vi "浊度电极校准.vi"() -> ()   [LabVIEW 2016, in "斯坦道多参数.lvlib"]
uses:
  <vilib>/Utility/miscctls.llb/LVPointTypeDef.ctl
  <vilib>/Utility/miscctls.llb/LVPositionTypeDef.ctl
  <vilib>/Analysis/NI_AALBase.lvlib
panel:
  out "滤波设定":dbl
  in  "刷新按钮":bool
  out "第三点信号值":dbl
  out "第二点信号值":dbl
  out "第一点信号值":dbl
  out "温度":dbl format="%#.2f"
  out "通讯状态":string
  out "电极状态标志":u16(ring) items=["OK"=0, "第一点校正通过"=1, "第二点校正通过"=2, "悬浮物两点校准第一点校正通过"=11, "悬浮物两点校准第二点校正通过"=12, "浊度三点校正第一点校正通过"=31, "浊度三点校正第二点校正通过"=32, "浊度三点校正第三点校正通过"=33]
  out "第三点校准值":dbl
  out "标液3":dbl
  out "第二点校准值":dbl
  out "第一点校准值":dbl
  in  "校准停止":bool
  in  "校准启动":bool
  in  "校准模式":u16(ring) items=["两点校准", "单点校准", "三点校准"]
  out "最小值":sgl format="%#.2f"
  out "最大值":sgl format="%#.2f"
  out "波形图表":sgl(graph) caption="历史曲线"
  out "mean":dbl caption="均值" format="%#.2f"
  out "standard deviation":dbl caption="标准差" format="%#.2f"
  out "变异系数":dbl format="%#.6f"
  out "测量值":dbl format="%#.2f"
  out "提示":string
  out "标液2":dbl
  out "标液1":dbl
  out "信号值":dbl format="%#.2f"
  out "偏移值补偿":dbl caption="浊度偏移修正值" format="%#.2f"
  out "电极斜率":dbl format="%#.6f"
  out "电极零点":dbl format="%#.6f"
  # "浊度电极设定"
  # "℃"
  # "NTU"
  # "%"
  # "请选择校准模式:"
  # "NTU"
  # "NTU"
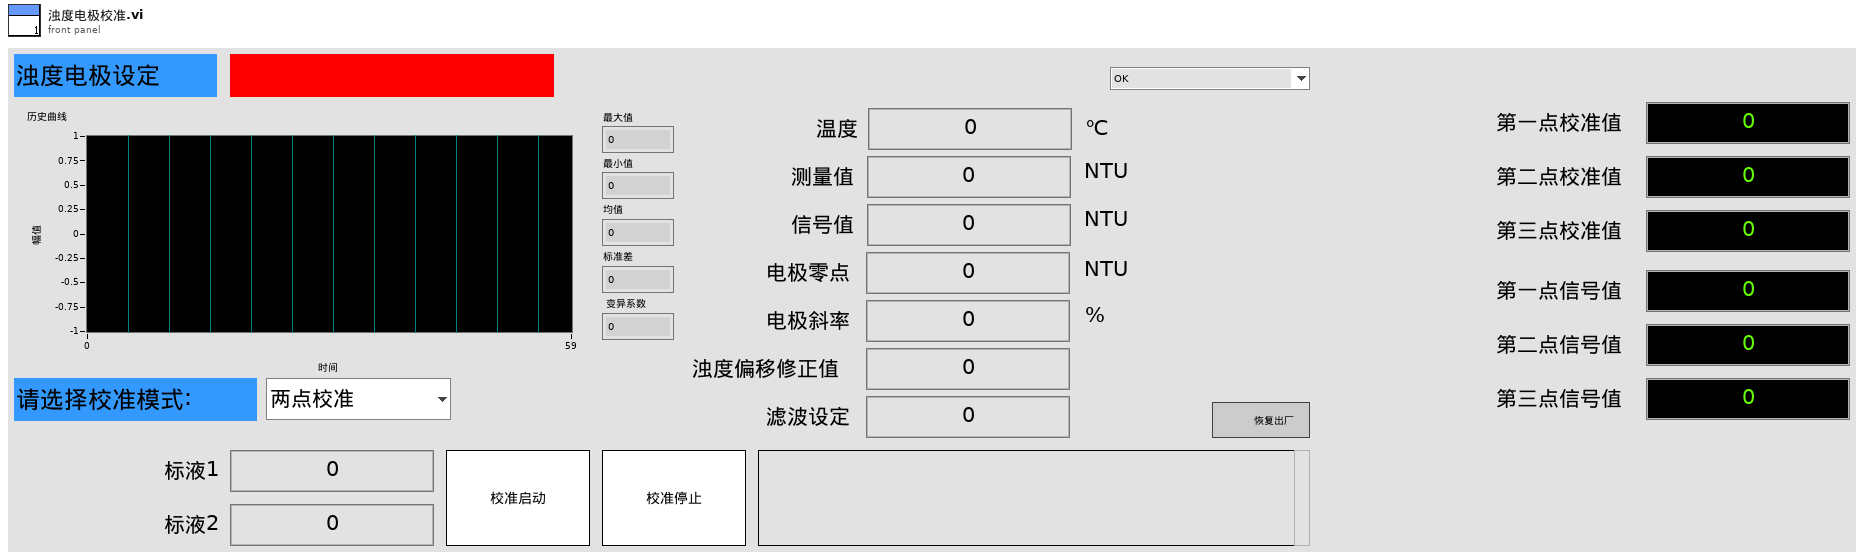
[diagram p1: front panel]
types:
  T1 = enum16{"pH", "DO", "Cond", "Turb", "ORP", "叶绿素a", "藻密度"}
  T2 = typedef "LVPointTypeDef.ctl" = cluster{"Horizontal":i16, "Vertical":i16}
  T3 = cluster{"电极状态标志":u16, "电极型号标志":u16, "浊度测量值":sgl, "温度测量值":sgl, "浊度信号值":sgl, "浊度偏移修正值":sgl, "温度偏移修正值":sgl, "手动温度补偿值":sgl, "浊度电极零点":sgl, "浊度电极斜率":sgl, "第1点标准值记录":sgl, "第1点信号值记录":sgl, "第1点温度值记录":sgl, "第2点标准值记录":sgl, "第2点信号值记录":sgl, "第2点温度值记录":sgl, "命令滤波设定":u16, "温度模式":enum16{"ATC", "MTC"}, "生产批次":u16, "电极序号":u16, "串口地址":u16, "串口波特率":enum16{"9600", "19200", "115200"}, "串口校验位":enum16{"NONE", "ODD", "EVEN"}, "串口停止位":enum16{"1bit", "2bit"}, "第一点标准值":sgl, "第二点标准值":sgl, "第三点标准值":sgl}
  T4 = typedef "LVPositionTypeDef.ctl" = cluster{"Left":i32, "Top":i32}
  T5 = enum8{"Enabled", "Disabled", "Disabled and Grayed Out"}
  T6 = cluster{"测量量程":dbl, "测量精度":dbl, "测量间隔":dbl, "消解温度":dbl, "消解时长":dbl, "空白校准时间":timestamp, "曲线截距":dbl, "曲线斜率":dbl, "测量检出限":dbl, "测量信号值":dbl, "线性相关系数":dbl, "二次多项式系数":dbl, "标样校准时间":timestamp, "稀释倍数":dbl, "三项式系数":dbl, "空白标定系数":dbl, "量程系数":dbl, "F0/ORPA":dbl, "F1/ORPB":dbl, "F2/ORPK":dbl, "F3":dbl, "F4":dbl, "F5":dbl, "F6":dbl, "F7":dbl, "X0/滴定数":dbl, "量程":dbl}
  T7 = cluster{"ph":bool, "DO":bool, "Cond":bool, "Turb":bool, "叶绿素a":bool, "藻密度":bool, "ORP":bool, "COD":bool}
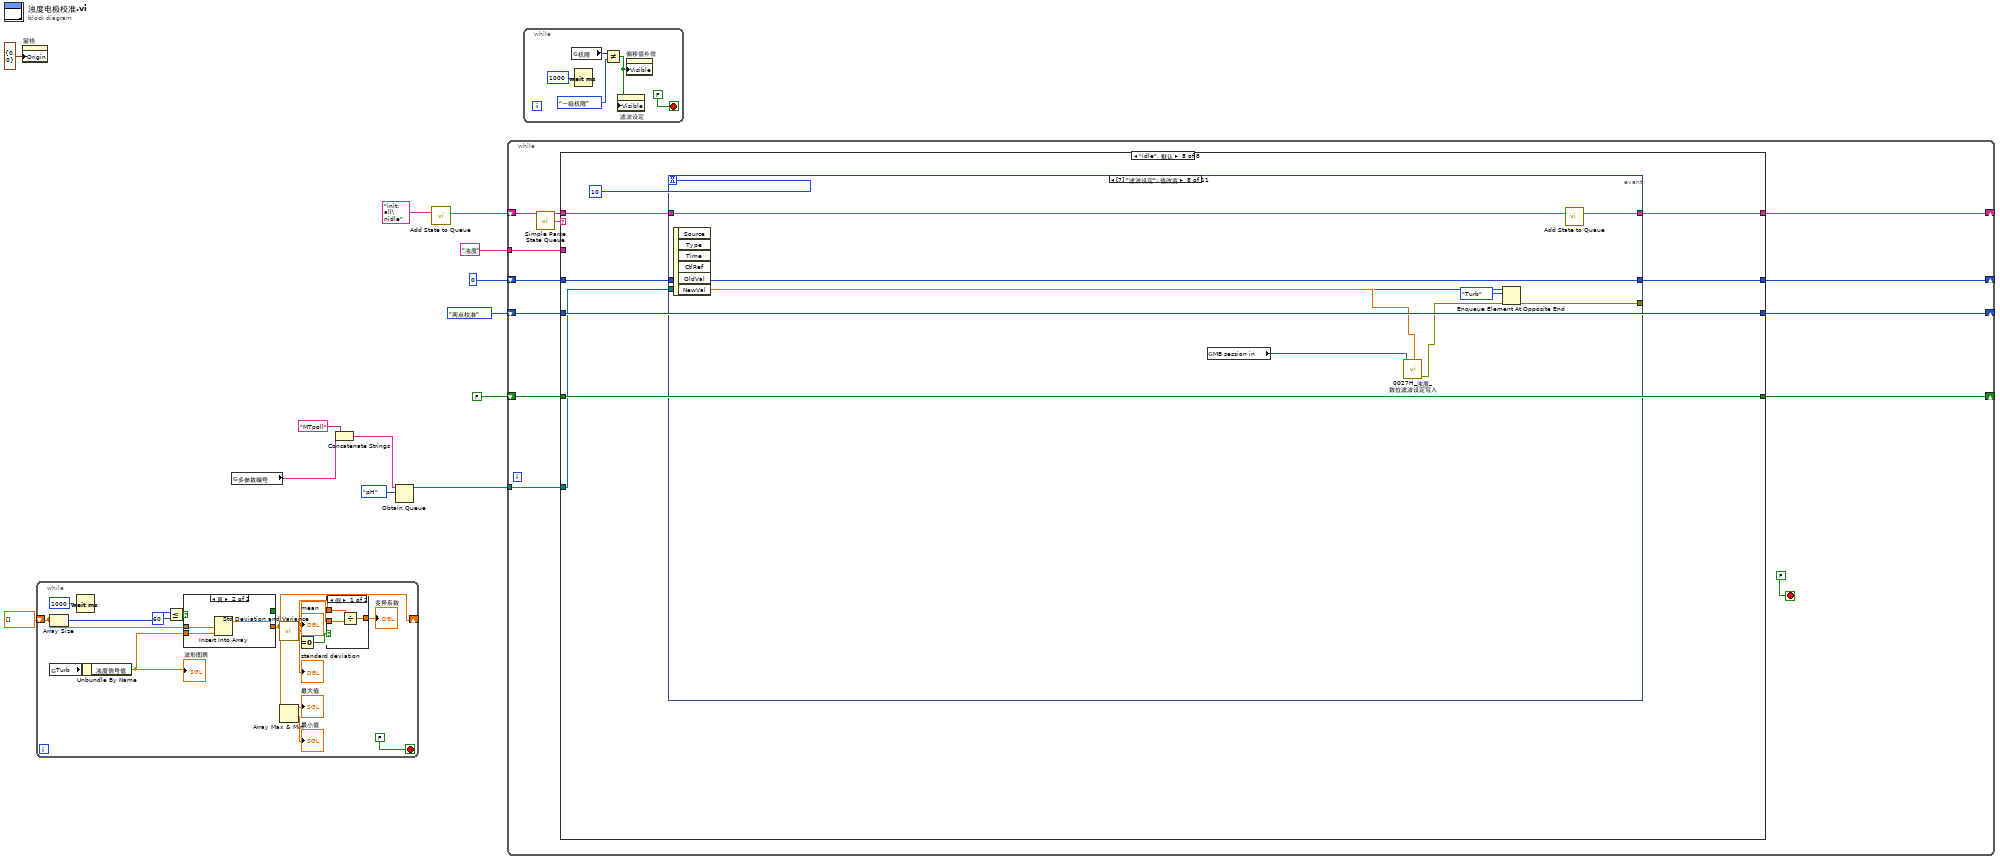
[diagram p0: block diagram]
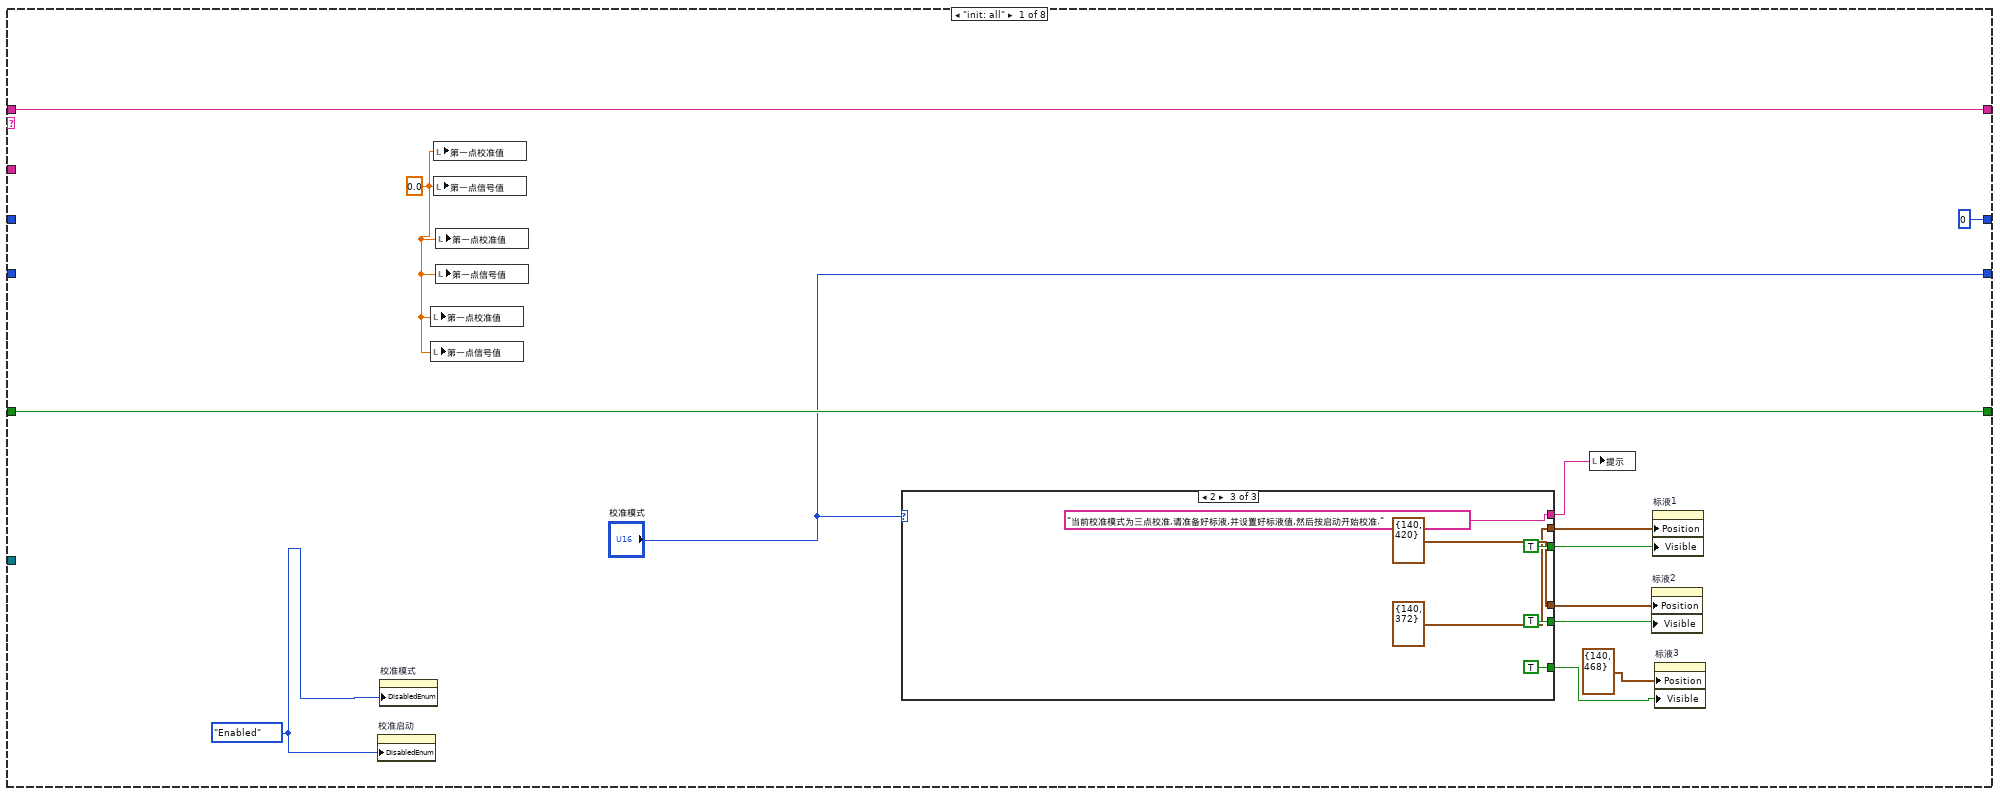
[diagram p2: hidden frame]
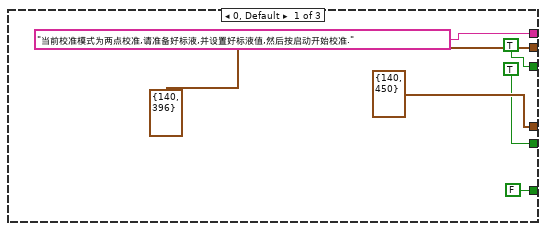
[diagram p3: hidden frame]
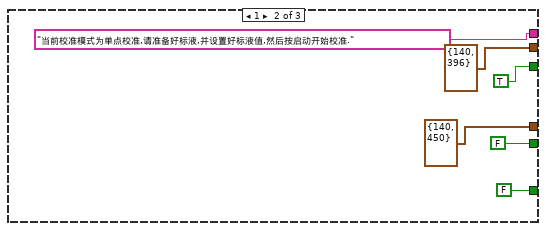
[diagram p4: hidden frame]
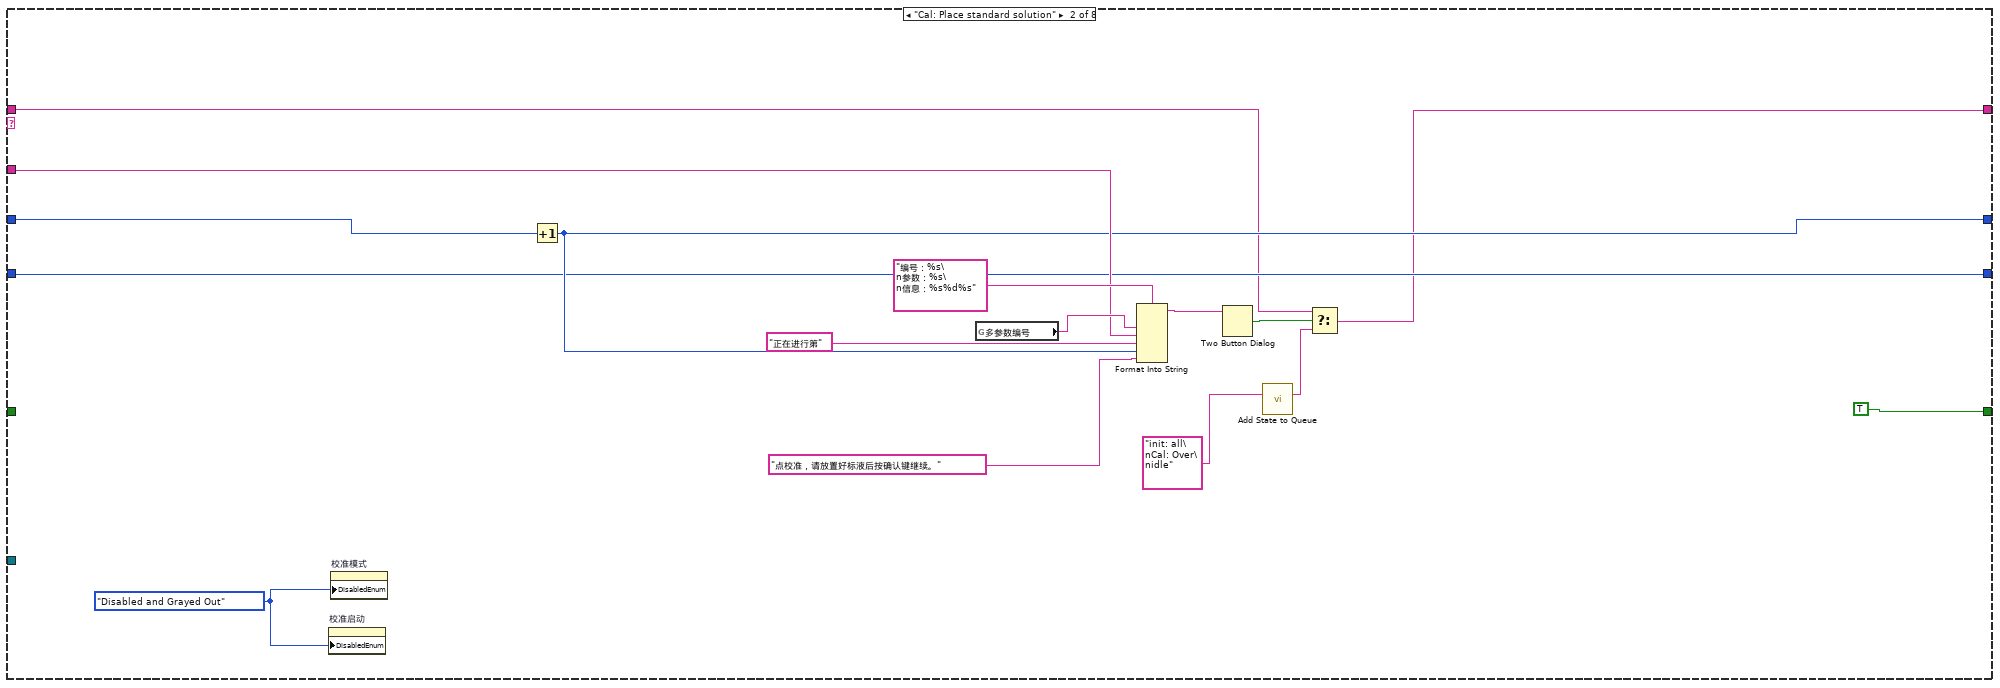
[diagram p5: hidden frame]
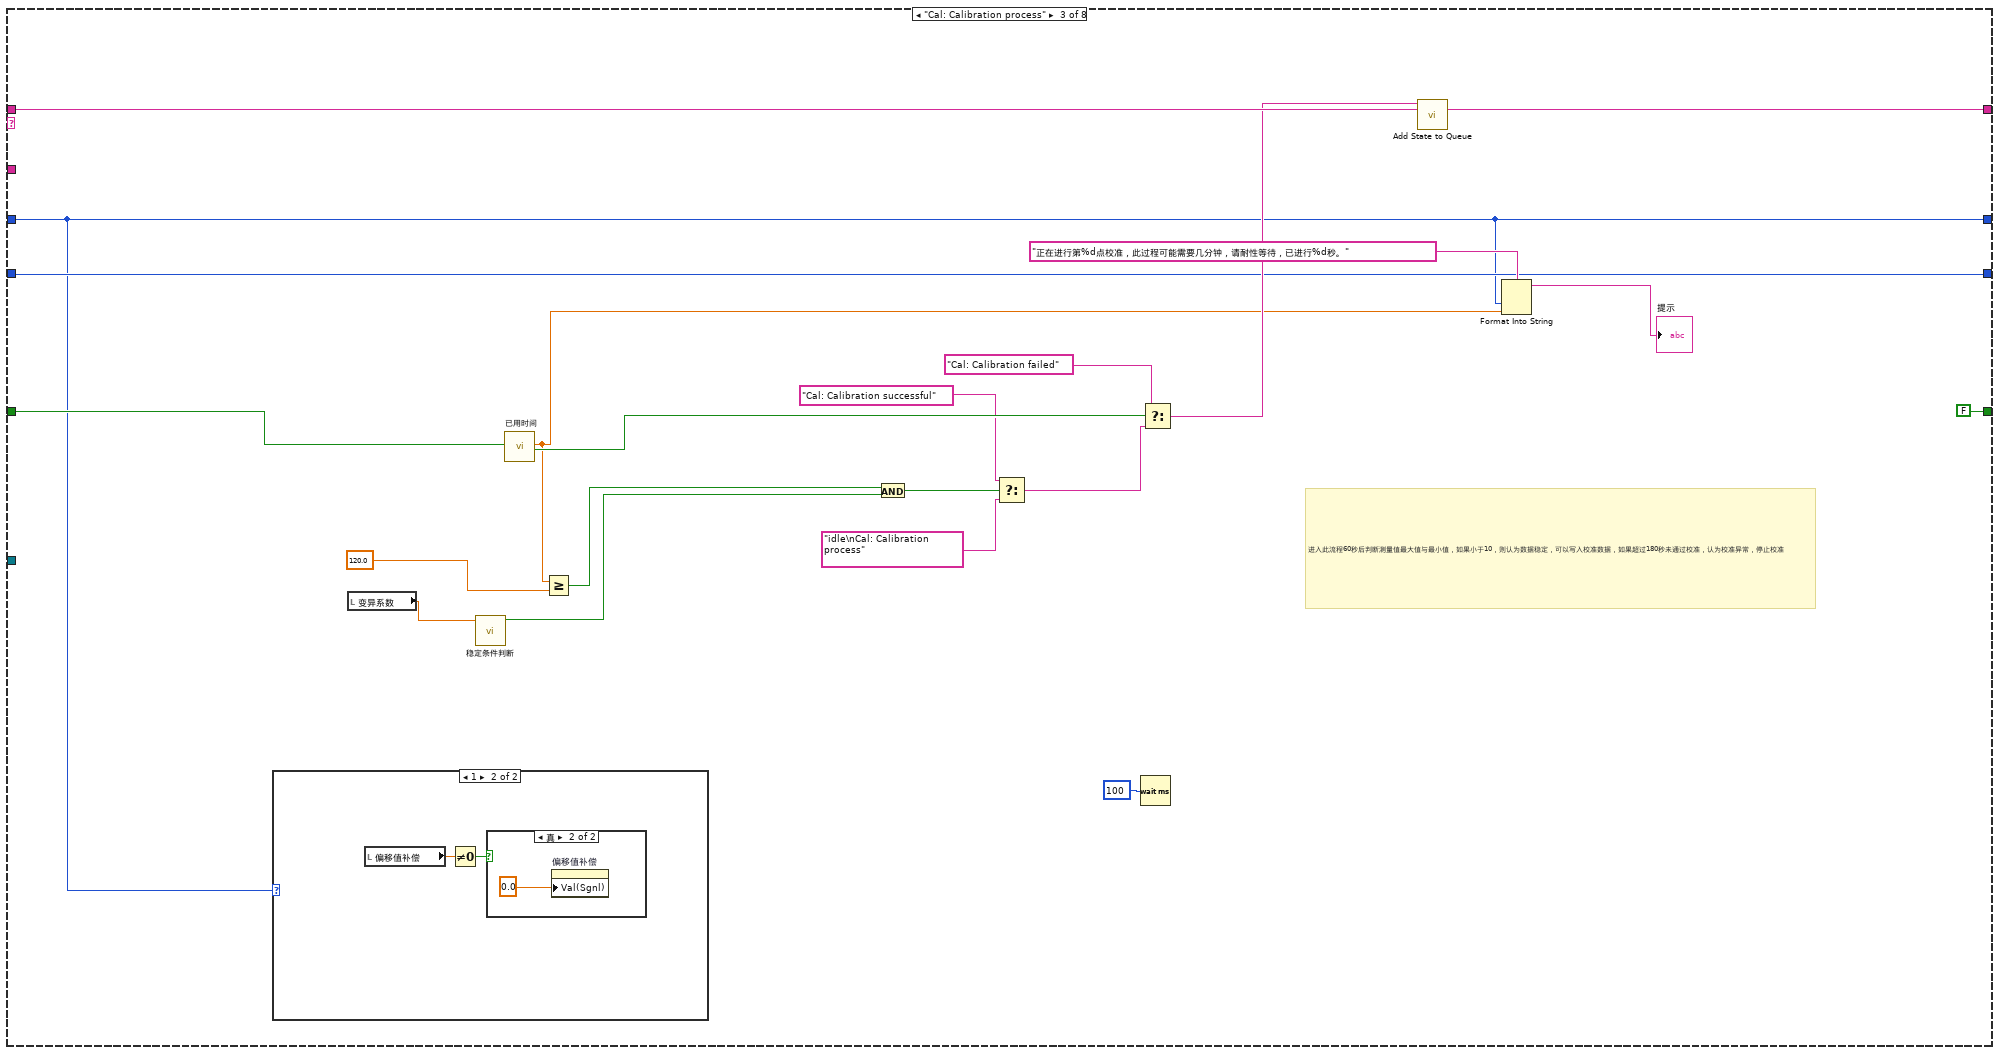
[diagram p6: hidden frame]
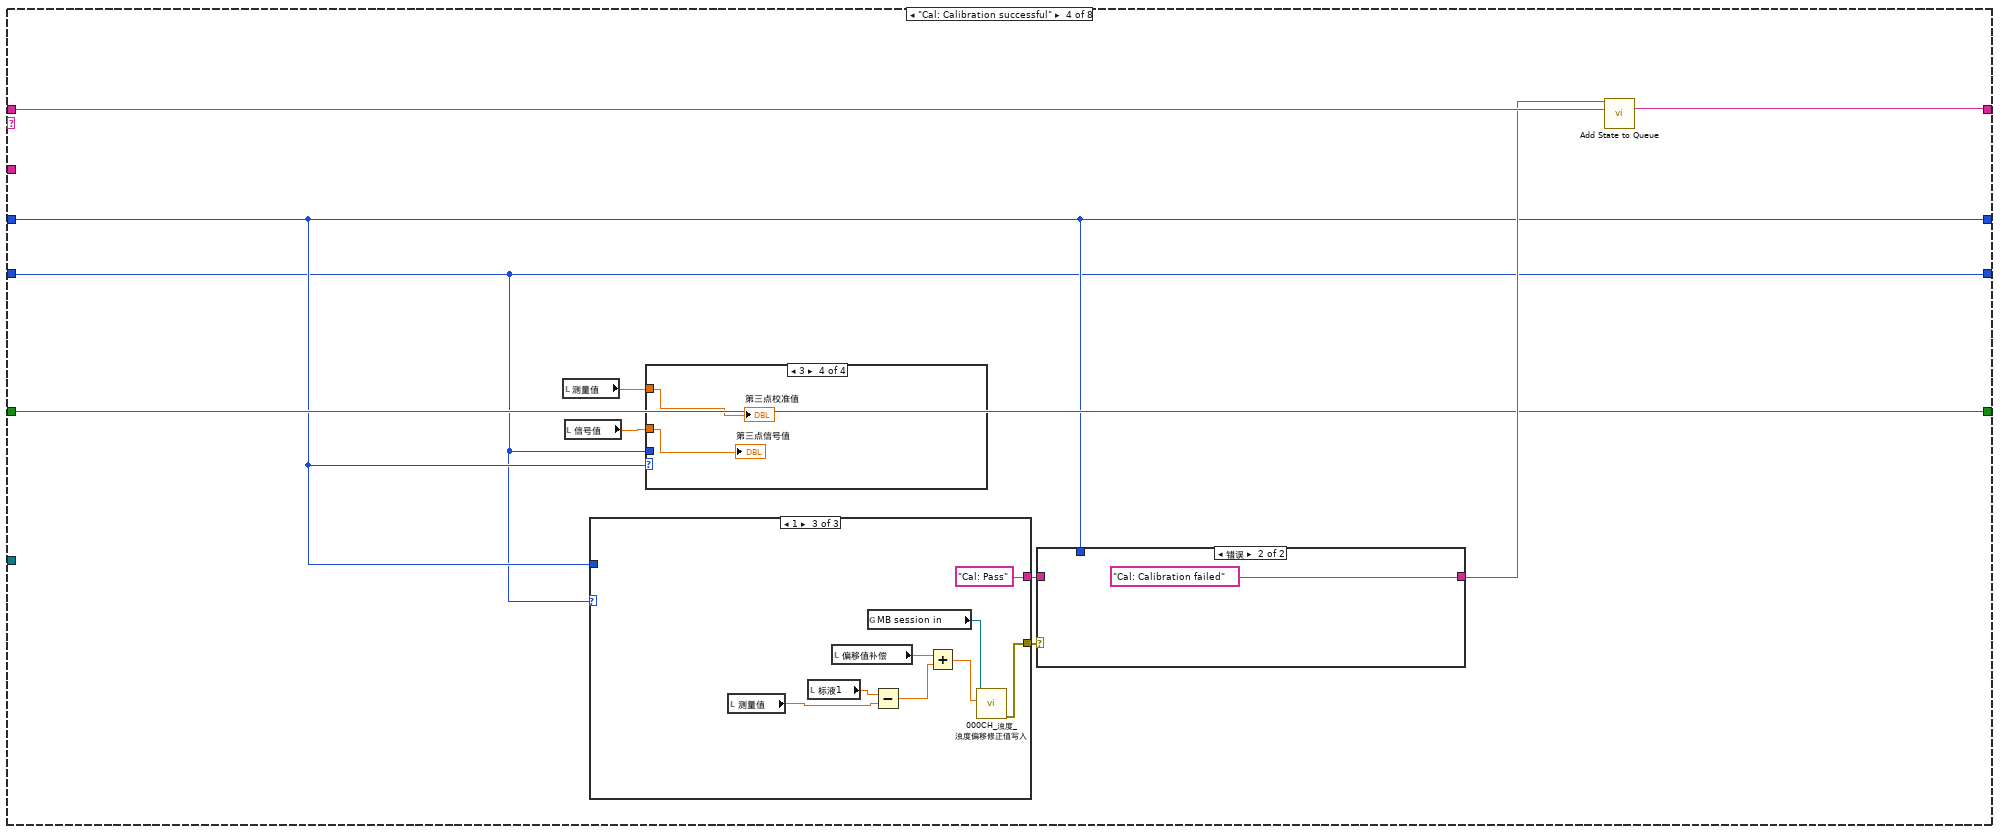
[diagram p9: hidden frame]
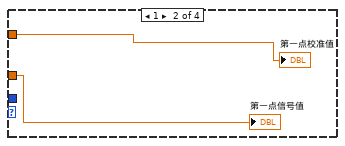
[diagram p11: hidden frame]
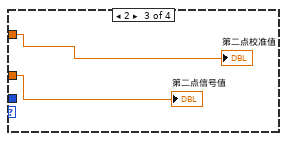
[diagram p12: hidden frame]
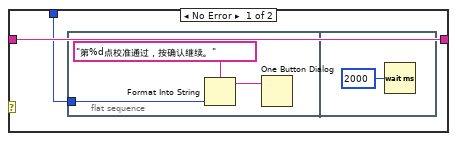
[diagram p13: hidden frame]
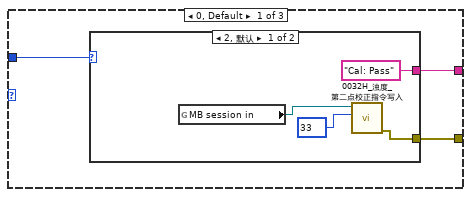
[diagram p14: hidden frame]
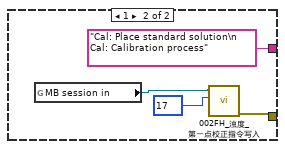
[diagram p15: hidden frame]
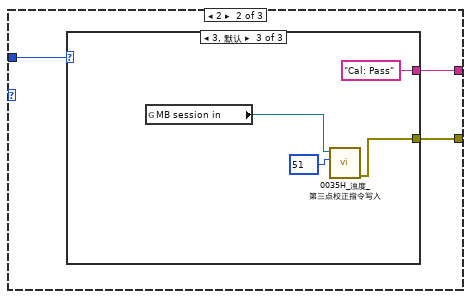
[diagram p16: hidden frame]
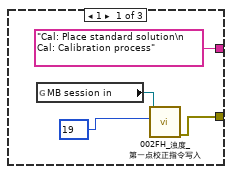
[diagram p17: hidden frame]
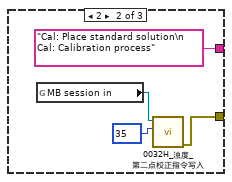
[diagram p18: hidden frame]
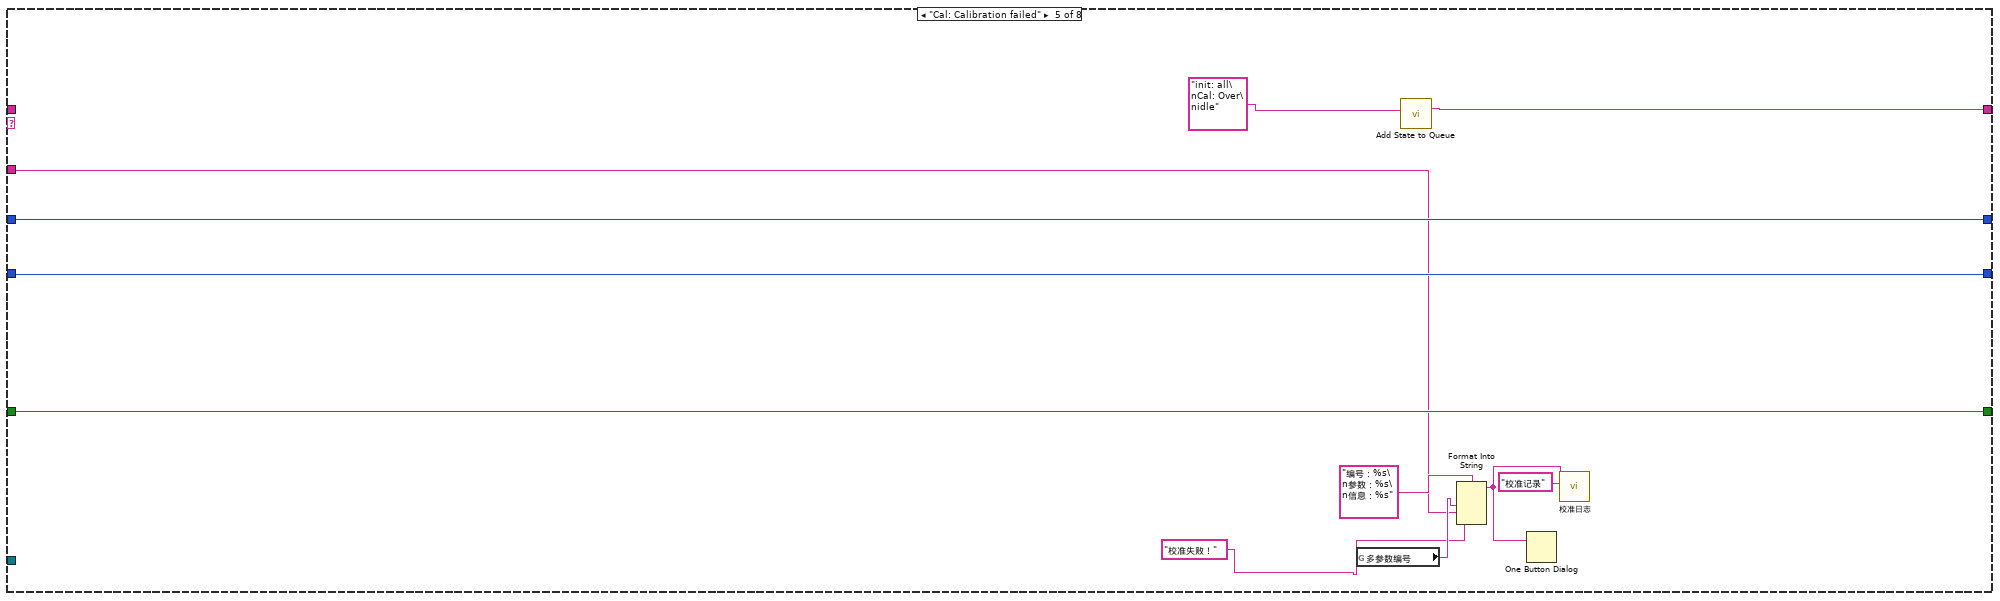
[diagram p19: hidden frame]
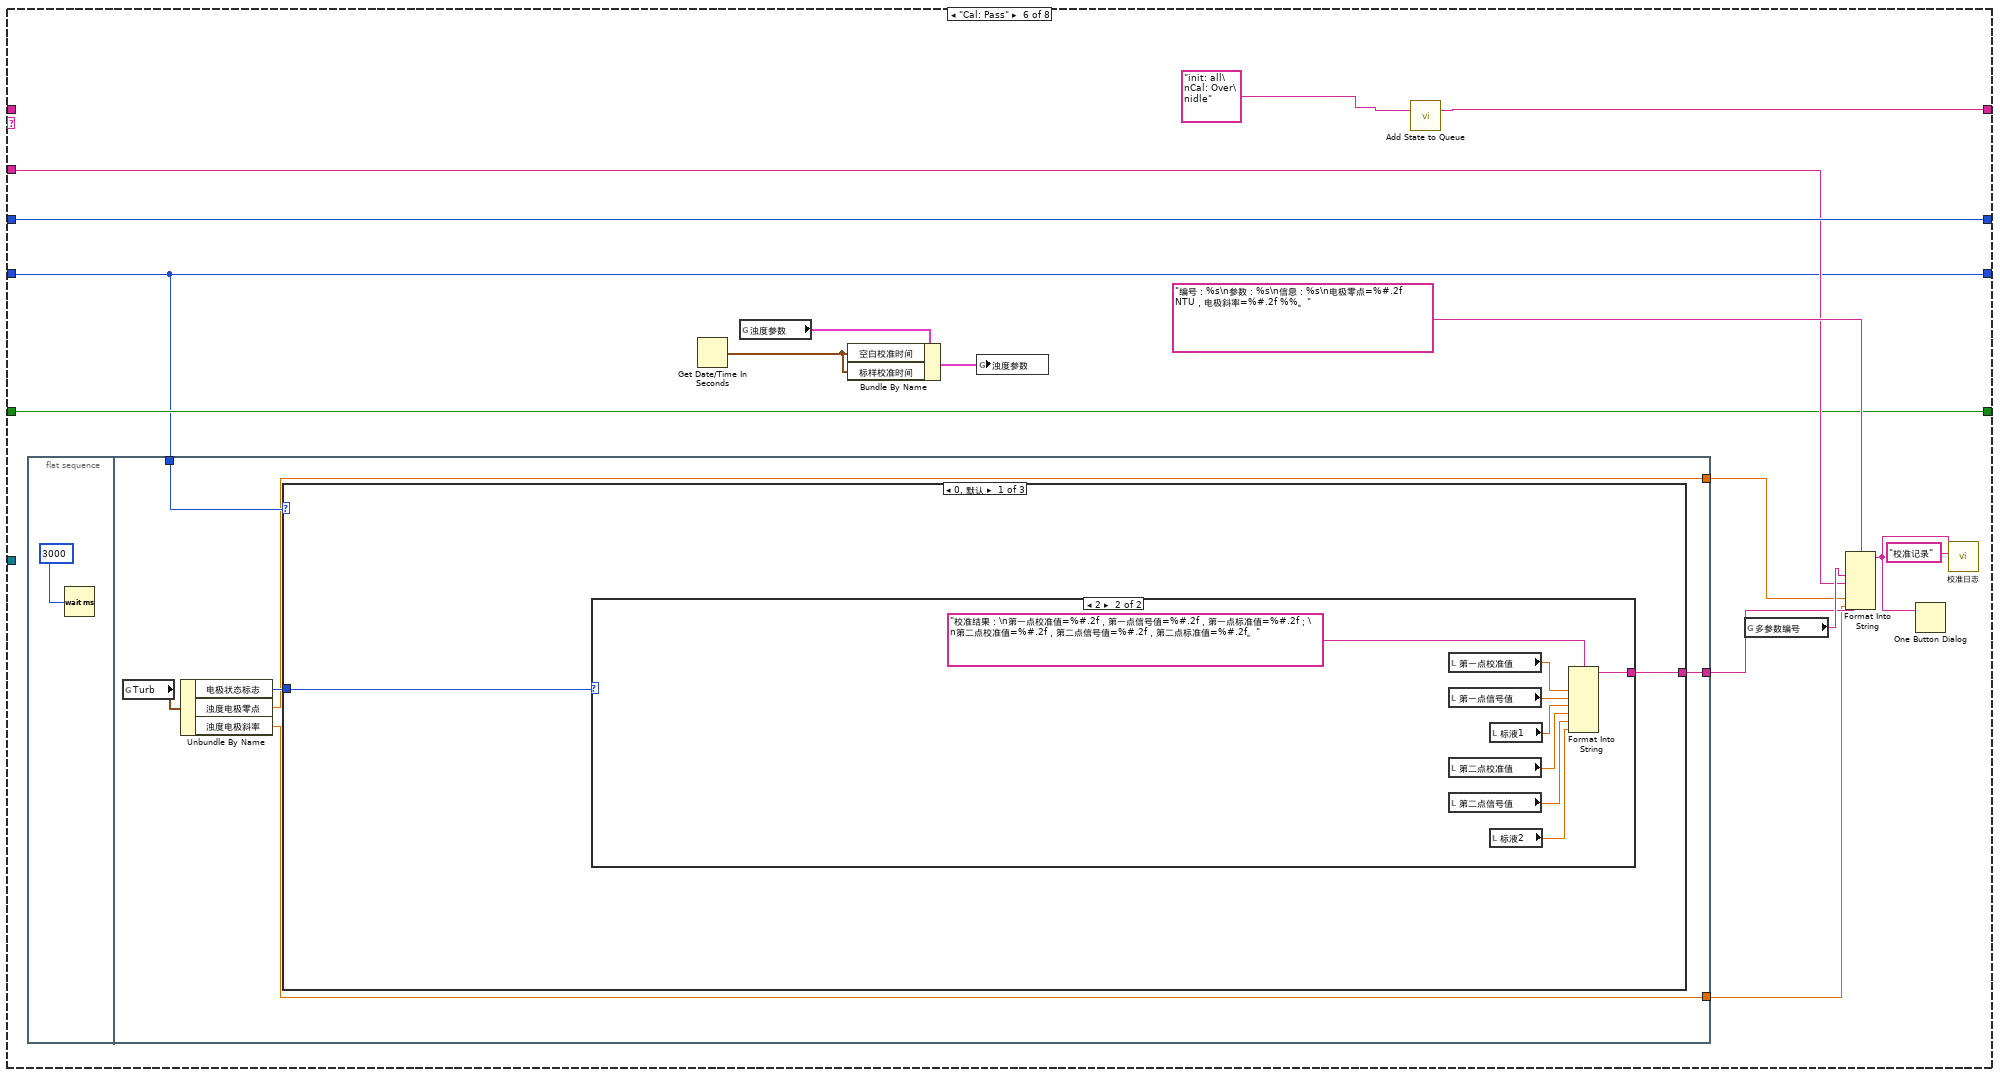
[diagram p20: hidden frame]
diagram:
  n1 = property on="窗格" class="Pane"("Origin"=T2 {"Horizontal"=0, "Vertical"=0} ("原点")) -> ()  [unwired: 2 in, 2 out]
  n2 = while {
    shift-right: [w17] -> _
    shift-left: sgl[] [] -> [w24]
    stop <- FALSE stop-if-true
    n3 = Array Size(array=w24) -> (size(s)=w26:i32)
    n4 = global read "国弘过程全局变量.vi" "Turb"() -> (w18:T3)
    n5 = Wait (ms)(milliseconds to wait=u32 1000 ("等待时间（毫秒）")) -> ()  [unwired: 1 out]
    n6 = Unbundle By Name(w18) -> ("浊度信号值"=w14:sgl)
    "波形图表" <- w14
    n7 = Less Or Equal?(x=w26, y=60) -> (x <= y?=w25:bool)
    n8 = case shown="真" w25 {
      tunnel: w24 -> [w37 w40]
      tunnel: w14 -> [w35 w39]
      tunnel: [w33 w38] -> w17
      tunnel: [TRUE _] -> _
      frame False {
        n9 = Replace Array Subset(array=w37, new element=w35) -> (w36:sgl[])  [unwired: 1 in]
        n10 = Rotate 1D Array(1:w36, 2:-1 ("n")) -> (0:w33:sgl[])
      }
      frame True {
        n11 = Insert Into Array(array=w40, new element=w39) -> (w38:sgl[])  [unwired: 1 in]
      }
    }
    n12 = call <vilib>:"Std Deviation and Variance.vi"("X"=w17) -> ("mean"=w22:dbl, "standard deviation"=w21:dbl)  [unwired: 1 in, 1 out]
    "mean" <- w22
    "standard deviation" <- w21
    n13 = Array Max & Min(array=w17) -> (max value=→"最大值":sgl, min value=→"最小值":sgl)  [unwired: 2 out]
    n14 = Equal To 0?(x=w22) -> (x = 0?=w23:bool)
    n15 = case shown="假" w23 {
      tunnel: w21 -> [w31 _]
      tunnel: [w30 _] -> w20
      tunnel: w22 -> [w29 _]
      frame False {
        n16 = Divide(x=w31, y=w29) -> (x/y=w30:dbl)
      }
      frame True {
      }
    }
    "变异系数" <- w20
  }
  n17 = global read "多参数全局变量.vi" "多参数编号"() -> (w2:string)
  n18 = Concatenate Strings("MTpoll" ("名称（未命名）"), w2) -> (w4:string)
  n19 = Obtain Queue(name (unnamed)=w4, element data type=T1."pH" ("枚举")) -> (queue out=w1:refnum<queue>)  [unwired: 3 in, 2 out]
  n20 = call "Add State to Queue.vi"("State(s) In (\"\")"="init: all\nidle" ("State(s) In (\"\")")) -> ("States Out"=w10:string)  [unwired: 14 in]
  n21 = while {
    shift-right: [w49] -> _
    shift-left: w10 -> [w53]
    shift-right: [w46] -> _
    shift-left: 0 -> [w48]
    tunnel: "浊度" ("State(s) In (\"\")") -> [w47]
    shift-right: [w44] -> _
    shift-left: enum16{"两点校准", "单点校准", "三点校准"}."两点校准" ("校准模式") -> [w45]
    shift-right: [w42] -> _
    shift-left: FALSE -> [w43]
    tunnel: w1 -> [w41]
    stop <- FALSE stop-if-true
    n22 = call "Simple Parse State Queue.vi"("State Queue"=w53) -> ("Remain States"=w50:string, "Next State"=w51:string)  [unwired: 13 in]
    n23 = case shown="\"idle\", 默认" w51 {
      tunnel: w50 -> [w66 w88 w120 w132 _ _ w249 w260]
      tunnel: [w66 w87 w119 w131 w189 w199 w249 w259] -> w49
      tunnel: w48 -> [_ w96 w105 w126 w192 w208 w248 w257]
      tunnel: w47 -> [_ w97 _ _ w183 w204 _ _]
      tunnel: [0 w94 w105 w126 w192 w208 w248 w258] -> w46
      tunnel: w45 -> [_ w93 w106 w125 w191 w200 w247 w256]
      tunnel: ["校准模式" w93 w106 w125 w191 w200 w247 w256] -> w44
      tunnel: w43 -> [w63 _ w108 w127 w190 w203 w246 w254]
      tunnel: [w63 TRUE FALSE w127 w190 w203 w246 w254] -> w42
      tunnel: w41 -> [_ _ _ _ _ _ _ w253]
      frame "init: all" {
        w61 = T5."Enabled" ("禁用")
        w62 = 0.0 ("第一点校准值")
        n24 = property on="校准启动" class="Bool"("DisabledEnum"=w61) -> ()  [unwired: 2 in, 2 out]
        n25 = property on="校准模式" class="Ring (严格)"("DisabledEnum"=w61) -> ()  [unwired: 2 in, 2 out]
        n26 = local write "第一点校准值"(w62) -> ()
        n27 = local write "第一点信号值"(w62) -> ()
        n28 = local write "第一点校准值"(w62) -> ()
        n29 = local write "第一点信号值"(w62) -> ()
        n30 = local write "第一点校准值"(w62) -> ()
        n31 = local write "第一点信号值"(w62) -> ()
        n32 = case shown="2" "校准模式" {
          tunnel: ["当前校准模式为两点校准,请准备好标液,并设置好标液值,然后按启动开始校准." ("提示") "当前校准模式为单点校准,请准备好标液,并设置好标液值,然后按启动开始校准." ("提示") "当前校准模式为三点校准,请准备好标液,并设置好标液值,然后按启动开始校准." ("提示")] -> w65
          tunnel: [T4 {"Left"=140, "Top"=396} ("位置") T4 {"Left"=140, "Top"=396} ("位置") T4 {"Left"=140, "Top"=372} ("位置")] -> w59
          tunnel: [TRUE ("可见") TRUE ("可见") TRUE ("可见")] -> w58
          tunnel: [FALSE ("可见") FALSE ("可见") TRUE ("可见")] -> w56
          tunnel: [TRUE ("可见") FALSE ("可见") TRUE ("可见")] -> w55
          tunnel: [T4 {"Left"=140, "Top"=450} ("位置 2") T4 {"Left"=140, "Top"=450} ("位置 2") T4 {"Left"=140, "Top"=420} ("位置 2")] -> w54
          frame 0, Default {
          }
          frame 1 {
          }
          frame 2 {
          }
        }
        n33 = local write "提示"(w65) -> ()
        n34 = property on="标液2" class="DigNum (严格)"("Position"=w54, "Visible"=w55) -> ()  [unwired: 2 in, 2 out]
        n35 = property on="标液1" class="DigNum (严格)"("Position"=w59, "Visible"=w58) -> ()  [unwired: 2 in, 2 out]
        n36 = property on="标液3" class="DigNum (严格)"("Position"=T4 {"Left"=140, "Top"=468} ("位置 3"), "Visible"=w56) -> ()  [unwired: 2 in, 2 out]
      }
      frame "Cal: Place standard solution" {
        w86 = T5."Disabled and Grayed Out" ("禁用")
        n37 = property on="校准启动" class="Bool"("DisabledEnum"=w86) -> ()  [unwired: 2 in, 2 out]
        n38 = property on="校准模式" class="Ring (严格)"("DisabledEnum"=w86) -> ()  [unwired: 2 in, 2 out]
        n39 = Increment(x=w96) -> (x+1=w94:i32)
        n40 = global read "多参数全局变量.vi" "多参数编号"() -> (w99:string)
        n41 = Format Into String(format string="编号：%s\n参数：%s\n信息：%s%d%s" ("格式字符串"), w99, w97, "正在进行第" ("消息"), w94, "点校准，请放置好标液后按确认键继续。" ("消息")) -> (resulting string=w91:string)  [unwired: 2 in, 1 out]
        n42 = Two Button Dialog(message=w91) -> (T button?=w90:bool)  [unwired: 2 in]
        n43 = call "Add State to Queue.vi"("State(s) In (\"\")"="init: all\nCal: Over\nidle" ("State(s) In (\"\")")) -> ("States Out"=w89:string)  [unwired: 14 in]
        n44 = Select(t=w88, s=w90, f=w89) -> (s? t:f=w87:string)
      }
      frame "Cal: Calibration process" {
        # "进入此流程60秒后判断测量值最大值与最小值，如果小于10，则认为数据稳定，可以写入校准数据，如果超过180秒未通过校准，认为校准异常，停止校准"
        n45 = case shown="1" w105 {
          frame 0, Default {
          }
          frame 1 {
            n46 = local read "偏移值补偿"() -> (w122:dbl)
            n47 = Not Equal To 0?(x=w122) -> (x != 0?=w123:bool)
            n48 = case shown="真" w123 {
              frame False {
              }
              frame True {
                n49 = property on="偏移值补偿" class="DigNum (严格)"("Val(Sgnl)"=0.0 ("值(信号)")) -> ()  [unwired: 2 in, 2 out]
              }
            }
          }
        }
        n50 = local read "变异系数"() -> (w102:dbl)
        n51 = call "稳定条件判断.vi"("变异系数"=w102) -> ("布尔"=w101:bool)  [unwired: 10 in]
        n52 = call "已用时间"("Reset"=w108) -> ("Elapsed Time (s)"=w104:dbl, "Time has Elapsed"=w121:bool)  [unwired: 11 in, 6 out]
        n53 = Greater Or Equal?(x=w104, y=120.0) -> (x >= y?=w116:bool)
        n54 = And(x=w116, y=w101) -> (x .and. y?=w113:bool)
        n55 = Select(t="Cal: Calibration successful" ("State(s) In (\"\")"), s=w113, f="idle\nCal: Calibration process" ("State(s) In (\"\")")) -> (s? t:f=w112:string)
        n56 = Wait (ms)(milliseconds to wait=u32 100 ("等待时间（毫秒）")) -> ()  [unwired: 1 out]
        n57 = Select(t="Cal: Calibration failed" ("State(s) In (\"\")"), s=w121, f=w112) -> (s? t:f=w111:string)
        n58 = call "Add State to Queue.vi"("State(s) In Front (\"\")"=w111, "State(s) In (\"\")"=w120) -> ("States Out"=w119:string)  [unwired: 13 in]
        n59 = Format Into String(format string="正在进行第%d点校准，此过程可能需要几分钟，请耐性等待，已进行%d秒。" ("格式字符串"), w105, w104) -> (resulting string=→"提示":string)  [unwired: 2 in, 1 out]
      }
      frame "Cal: Calibration successful" {
        n60 = local read "测量值"() -> (w128:dbl)
        n61 = local read "信号值"() -> (w129:dbl)
        n62 = case shown="1" w125 {
          tunnel: [w150 w161 w174] -> w134
          tunnel: [w149 w159 "Cal: Pass" ("State(s) In (\"\")")] -> w133
          tunnel: w126 -> [w148 w160 _]
          frame 0, Default {
            n63 = case shown="2, 默认" w148 {
              tunnel: [w153 w157] -> w150
              tunnel: ["Cal: Pass" ("State(s) In (\"\")") "Cal: Place standard solution\n Cal: Calibration process" ("State(s) In (\"\")")] -> w149
              frame 2, Default {
                n64 = global read "多参数全局变量.vi" "MB session in"() -> (w152:refnum<class "MB_Master.lvclass">)
                n65 = call "0032H_浊度_第二点校正指令写入.vi"("数值"=u16 33, "MB session in"=w152) -> ("error out"=w153:errorcluster)  [unwired: 8 in, 1 out]
              }
              frame 1 {
                n66 = global read "多参数全局变量.vi" "MB session in"() -> (w156:refnum<class "MB_Master.lvclass">)
                n67 = call "002FH_浊度_第一点校正指令写入.vi"("数值"=u16 17, "MB session in"=w156) -> ("error out"=w157:errorcluster)  [unwired: 8 in, 1 out]
              }
            }
          }
          frame 2 {
            n68 = case shown="3, 默认" w160 {
              tunnel: [w164 w167 w171] -> w161
              tunnel: ["Cal: Place standard solution\n Cal: Calibration process" ("State(s) In (\"\")") "Cal: Place standard solution\n Cal: Calibration process" ("State(s) In (\"\")") "Cal: Pass" ("State(s) In (\"\")")] -> w159
              frame 1 {
                n69 = global read "多参数全局变量.vi" "MB session in"() -> (w163:refnum<class "MB_Master.lvclass">)
                n70 = call "002FH_浊度_第一点校正指令写入.vi"("数值"=u16 19, "MB session in"=w163) -> ("error out"=w164:errorcluster)  [unwired: 8 in, 1 out]
              }
              frame 2 {
                n71 = global read "多参数全局变量.vi" "MB session in"() -> (w166:refnum<class "MB_Master.lvclass">)
                n72 = call "0032H_浊度_第二点校正指令写入.vi"("数值"=u16 35, "MB session in"=w166) -> ("error out"=w167:errorcluster)  [unwired: 8 in, 1 out]
              }
              frame 3, Default {
                n73 = global read "多参数全局变量.vi" "MB session in"() -> (w170:refnum<class "MB_Master.lvclass">)
                n74 = call "0035H_浊度_第三点校正指令写入.vi"("数值"=u16 51, "MB session in"=w170) -> ("error out"=w171:errorcluster)  [unwired: 8 in, 1 out]
              }
            }
          }
          frame 1 {
            n75 = local read "测量值"() -> (w177:dbl)
            n76 = local read "标液1"() -> (w181:dbl)
            n77 = local read "偏移值补偿"() -> (w179:dbl)
            n78 = global read "多参数全局变量.vi" "MB session in"() -> (w176:refnum<class "MB_Master.lvclass">)
            n79 = Subtract(x=w181, y=w177) -> (x-y=w180:dbl)
            n80 = Add(x=w179, y=w180) -> (x+y=w175:dbl)
            n81 = call "000CH_浊度_浊度偏移修正值写入.vi"("数值"=w175, "MB session in"=w176) -> ("error out"=w174:errorcluster)  [unwired: 8 in, 1 out]
          }
        }
        n82 = case shown="3" w126 {
          tunnel: w129 -> [_ w136 w138 w140]
          tunnel: w128 -> [_ w135 w137 w139]
          tunnel: w125 -> [_ _ _ _]
          frame 0, Default {
          }
          frame 1 {
            "第一点信号值" <- w136
            "第一点校准值" <- w135
          }
          frame 2 {
            "第二点信号值" <- w138
            "第二点校准值" <- w137
          }
          frame 3 {
            "第三点信号值" <- w140
            "第三点校准值" <- w139
          }
        }
        n83 = case shown="错误" w134 {
          tunnel: w133 -> [w142 _]
          tunnel: [w142 "Cal: Calibration failed" ("State(s) In (\"\")")] -> w130
          tunnel: w126 -> [w141 _]
          frame No Error {
            n84 = flat-sequence {
              tunnel: w141 -> [w143]
              frame #0 {
                n85 = Format Into String(format string="第%d点校准通过，按确认继续。" ("格式字符串"), w143) -> (resulting string=w145:string)  [unwired: 2 in, 1 out]
                n86 = One Button Dialog(message=w145) -> ()  [unwired: 1 in, 1 out]
              }
              frame #1 {
                n87 = Wait (ms)(milliseconds to wait=u32 2000 ("等待时间（毫秒）")) -> ()  [unwired: 1 out]
              }
            }
          }
          frame Error {
          }
        }
        n88 = call "Add State to Queue.vi"("State(s) In Front (\"\")"=w130, "State(s) In (\"\")"=w132) -> ("States Out"=w131:string)  [unwired: 13 in]
      }
      frame "Cal: Calibration failed" {
        n89 = global read "多参数全局变量.vi" "多参数编号"() -> (w186:string)
        n90 = call "Add State to Queue.vi"("State(s) In (\"\")"="init: all\nCal: Over\nidle" ("State(s) In (\"\")")) -> ("States Out"=w189:string)  [unwired: 14 in]
        n91 = Format Into String(format string="编号：%s\n参数：%s\n信息：%s" ("格式字符串"), w186, w183, "校准失败！" ("消息")) -> (resulting string=w185:string)  [unwired: 2 in, 1 out]
        n92 = One Button Dialog(message=w185) -> ()  [unwired: 1 in, 1 out]
        n93 = call "校准日志.vi"("table"="校准记录", "日志信息"=w185) -> ()  [unwired: 9 in, 1 out]
      }
      frame "Cal: Pass" {
        n94 = flat-sequence {
          tunnel: [w213] -> w201
          tunnel: w200 -> [w212]
          tunnel: [w211] -> w198
          tunnel: [w210] -> w197
          frame #0 {
            n95 = Wait (ms)(milliseconds to wait=u32 3000 ("等待时间（毫秒）")) -> ()  [unwired: 1 out]
          }
          frame #1 {
            n96 = global read "国弘过程全局变量.vi" "Turb"() -> (w214:T3)
            n97 = Unbundle By Name(w214) -> ("电极状态标志"=w215:u16, "浊度电极零点"=w211:sgl, "浊度电极斜率"=w210:sgl)
            n98 = case shown="0, 默认" w212 {
              tunnel: [w217 w228 w245] -> w213
              tunnel: w215 -> [w216 w227 _]
              frame 0, Default {
                n99 = case shown="2" w216 {
                  tunnel: ["校准异常，校准未完成。" ("格式字符串") w226] -> w217
                  frame 0, Default {
                  }
                  frame 2 {
                    n100 = local read "第一点校准值"() -> (w224:dbl)
                    n101 = local read "第一点信号值"() -> (w225:dbl)
                    n102 = local read "第二点校准值"() -> (w221:dbl)
                    n103 = local read "第二点信号值"() -> (w220:dbl)
                    n104 = local read "标液1"() -> (w222:dbl)
                    n105 = local read "标液2"() -> (w219:dbl)
                    n106 = Format Into String(format string="校准结果：\n第一点校准值=%#.2f，第一点信号值=%#.2f，第一点标准值=%#.2f；\n第二点校准值=%#.2f，第二点信号值=%#.2f，第二点标准值=%#.2f。" ("提示"), w224, w225, w222, w221, w220, w219) -> (resulting string=w226:string)  [unwired: 2 in, 1 out]
                  }
                }
              }
              frame 2 {
                n107 = case shown="33" w227 {
                  tunnel: ["校准异常，校准未完成。" ("格式字符串") w240] -> w228
                  frame 0, Default {
                  }
                  frame 33 {
                    n108 = local read "标液2"() -> (w231:dbl)
                    n109 = local read "标液1"() -> (w232:dbl)
                    n110 = local read "第一点校准值"() -> (w239:dbl)
                    n111 = local read "第一点信号值"() -> (w237:dbl)
                    n112 = local read "第二点校准值"() -> (w236:dbl)
                    n113 = local read "第二点信号值"() -> (w235:dbl)
                    n114 = local read "第三点校准值"() -> (w234:dbl)
                    n115 = local read "第三点信号值"() -> (w233:dbl)
                    n116 = local read "标液3"() -> (w230:dbl)
                    n117 = Format Into String(format string="校准结果：\n第一点校准值=%#.2f，第一点信号值=%#.2f，第一点标准值=%#.2f；\n第二点校准值=%#.2f，第二点信号值=%#.2f，第二点标准值=%#.2f；\n第三点校准值=%#.2f，第三点信号值=%#.2f，第三点标准值=%#.2f。" ("提示"), w239, w237, w232, w236, w235, w231, w234, w233, w230) -> (resulting string=w240:string)  [unwired: 2 in, 1 out]
                  }
                }
              }
              frame 1 {
                n118 = local read "第一点校准值"() -> (w244:dbl)
                n119 = local read "第一点信号值"() -> (w242:dbl)
                n120 = local read "标液1"() -> (w241:dbl)
                n121 = Format Into String(format string="校准结果：\n校准值=%#.2f，信号值=%#.2f，标准值=%#.2f。" ("提示"), w244, w242, w241) -> (resulting string=w245:string)  [unwired: 2 in, 1 out]
              }
            }
          }
        }
        n122 = Get Date/Time In Seconds() -> (seconds since 1Jan1904=w193:timestamp)
        n123 = global read "断电保存变量.vi" "浊度参数"() -> (w195:T6)
        n124 = Bundle By Name(cluster=w195, "空白校准时间"=w193, "标样校准时间"=w193) -> (w194:T6)
        n125 = global write "断电保存变量.vi" "浊度参数"(w194) -> ()
        n126 = call "Add State to Queue.vi"("State(s) In (\"\")"="init: all\nCal: Over\nidle" ("State(s) In (\"\")")) -> ("States Out"=w199:string)  [unwired: 14 in]
        n127 = global read "多参数全局变量.vi" "多参数编号"() -> (w205:string)
        n128 = Format Into String(format string="编号：%s\n参数：%s\n信息：%s\n电极零点=%#.2f NTU，电极斜率=%#.2f %%。" ("格式字符串"), w205, w204, w201, w198, w197) -> (resulting string=w202:string)  [unwired: 2 in, 1 out]
        n129 = One Button Dialog(message=w202) -> ()  [unwired: 1 in, 1 out]
        n130 = call "校准日志.vi"("table"="校准记录", "日志信息"=w202) -> ()  [unwired: 9 in, 1 out]
      }
      frame "Cal: Over" {
        n131 = global read "多参数全局变量.vi" "校准运行状态"() -> (w251:T7)
        n132 = Bundle By Name(cluster=w251, "Turb"=FALSE) -> (w252:T7)
        n133 = global write "多参数全局变量.vi" "校准运行状态"(w252) -> ()
      }
      frame "idle", Default {
        n134 = event shown="[7] \"滤波设定\": 值改变" {
          selector: _ -> [_ _ _ _ _ _ _ _ _ _ _]
          dyn-events: _ -> [_ _ _ _ _ _ _ _ _ _ _]
          timeout: 10 -> [_ _ _ _ _ _ _ _ _ _ _]
          tunnel: [_ _ _ w293 w302 w311 w320 w329 _ _ _] -> _
          tunnel: w260 -> [w279 w283 w288 w299 w303 w312 w321 w333 w340 w349 _]
          tunnel: [w278 w282 w289 w298 w307 w316 w325 w334 w339 w348 w351] -> w259
          tunnel: [w277 w280 w290 w297 w308 w317 w326 w335 w338 w346 w352] -> w258
          tunnel: w257 -> [w277 w280 w290 w297 w308 w317 w326 w335 w338 w346 w352]
          tunnel: w253 -> [_ _ _ w292 w301 w310 w319 w328 _ _ _]
          event Timeout {
            n135 = event-data() -> ()  [unwired: 1 in, 3 out]
            n136 = global read "国弘过程全局变量.vi" "Turb"() -> (w262:T3)
            n137 = Unbundle By Name(w262) -> ("命令滤波设定"=→"滤波设定":u16, "电极状态标志"=→"电极状态标志":u16, "浊度电极零点"=→"电极零点":sgl, "浊度电极斜率"=→"电极斜率":sgl, "浊度偏移修正值"=→"偏移值补偿":sgl, "浊度信号值"=→"信号值":sgl, "第一点标准值"=→"标液1":sgl, "第二点标准值"=→"标液2":sgl, "浊度测量值"=→"测量值":sgl, "第三点标准值"=→"标液3":sgl, "温度测量值"=→"温度":sgl)  [unwired: 1 out]
            n138 = global read "多参数全局变量.vi" "浊度通讯状态"() -> (w274:bool)
            n139 = property on="通讯状态" class="Str"("Blinking"=TRUE ("闪烁"), "Text.BG Color"=u32 16711680, "Visible"=w274) -> ()  [unwired: 2 in, 2 out]
            n140 = call "Add State to Queue.vi"("State(s) In (\"\")"=w279) -> ("States Out"=w278:string)  [unwired: 14 in]
            "通讯状态" <- "通讯异常" ("当前串口")
          }
          event "校准模式": Value Change {
            n141 = event-data() -> ()  [unwired: 1 in, 6 out]
            n142 = call "Add State to Queue.vi"("State(s) In (\"\")"=w283, "State(s) At Back (\"\")"="init: all\nidle" ("State(s) In (\"\")")) -> ("States Out"=w282:string)  [unwired: 13 in]
          }
          event "偏移值补偿", "标液1", "标液2", "标液3", "滤波设定": Mouse Down {
            n143 = event-data() -> ("CtlRef"=w287:refnum<vi>)  [unwired: 1 in, 7 out]
            n144 = property class="DigNum (严格)"(reference=w287) -> (reference out=w284:refnum<vi>, "Value"=w285:dbl)  [unwired: 1 in, 1 out]
            n145 = call "数字键盘.vi"("OldNumber"=w285) -> ("NewNumber"=w286:dbl)  [unwired: 1 in]
            n146 = property class="DigNum (严格)"(reference=w284, "Val(Sgnl)"=w286) -> ()  [unwired: 1 in, 2 out]
            n147 = call "Add State to Queue.vi"("State(s) In (\"\")"=w288) -> ("States Out"=w289:string)  [unwired: 14 in]
          }
          event "偏移值补偿": Value Change {
            n148 = event-data() -> ("NewVal"=w294:dbl)  [unwired: 1 in, 5 out]
            n149 = global read "多参数全局变量.vi" "MB session in"() -> (w295:refnum<class "MB_Master.lvclass">)
            n150 = call "000CH_浊度_浊度偏移修正值写入.vi"("数值"=w294, "MB session in"=w295) -> ("error out"=w296:errorcluster)  [unwired: 8 in, 1 out]
            n151 = Enqueue Element At Opposite End(queue=w292, element=T1."Turb" ("元素"), error in (no error)=w296) -> (error out=w293:errorcluster)  [unwired: 1 in, 2 out]
            n152 = call "Add State to Queue.vi"("State(s) In (\"\")"=w299) -> ("States Out"=w298:string)  [unwired: 14 in]
          }
          event "标液1": Value Change {
            n153 = event-data() -> ("NewVal"=w304:dbl)  [unwired: 1 in, 5 out]
            n154 = global read "多参数全局变量.vi" "MB session in"() -> (w305:refnum<class "MB_Master.lvclass">)
            n155 = call "0030H_浊度_第一点标准值写入.vi"("数值"=w304, "MB session in"=w305) -> ("error out"=w306:errorcluster)  [unwired: 8 in, 1 out]
            n156 = Enqueue Element At Opposite End(queue=w301, element=T1."Turb" ("元素"), error in (no error)=w306) -> (error out=w302:errorcluster)  [unwired: 1 in, 2 out]
            n157 = call "Add State to Queue.vi"("State(s) In (\"\")"=w303) -> ("States Out"=w307:string)  [unwired: 14 in]
          }
          event "标液2": Value Change {
            n158 = event-data() -> ("NewVal"=w313:dbl)  [unwired: 1 in, 5 out]
            n159 = global read "多参数全局变量.vi" "MB session in"() -> (w314:refnum<class "MB_Master.lvclass">)
            n160 = call "0033H_浊度_第二点标准值写入.vi"("数值"=w313, "MB session in"=w314) -> ("error out"=w315:errorcluster)  [unwired: 8 in, 1 out]
            n161 = Enqueue Element At Opposite End(queue=w310, element=T1."Turb" ("元素"), error in (no error)=w315) -> (error out=w311:errorcluster)  [unwired: 1 in, 2 out]
            n162 = call "Add State to Queue.vi"("State(s) In (\"\")"=w312) -> ("States Out"=w316:string)  [unwired: 14 in]
          }
          event "标液3": Value Change {
            n163 = event-data() -> ("NewVal"=w322:dbl)  [unwired: 1 in, 5 out]
            n164 = global read "多参数全局变量.vi" "MB session in"() -> (w323:refnum<class "MB_Master.lvclass">)
            n165 = call "0036H_浊度_第三点标准值写入.vi"("数值"=w322, "MB session in"=w323) -> ("error out"=w324:errorcluster)  [unwired: 8 in, 1 out]
            n166 = Enqueue Element At Opposite End(queue=w319, element=T1."Turb" ("元素"), error in (no error)=w324) -> (error out=w320:errorcluster)  [unwired: 1 in, 2 out]
            n167 = call "Add State to Queue.vi"("State(s) In (\"\")"=w321) -> ("States Out"=w325:string)  [unwired: 14 in]
          }
          event "滤波设定": Value Change {
            n168 = event-data() -> ("NewVal"=w331:dbl)  [unwired: 1 in, 5 out]
            n169 = global read "多参数全局变量.vi" "MB session in"() -> (w332:refnum<class "MB_Master.lvclass">)
            n170 = call "0027H_浊度_数位滤波设定写入.vi"("数值"=w331, "MB session in"=w332) -> ("error out"=w330:errorcluster)  [unwired: 8 in, 1 out]
            n171 = Enqueue Element At Opposite End(queue=w328, element=T1."Turb" ("元素"), error in (no error)=w330) -> (error out=w329:errorcluster)  [unwired: 1 in, 2 out]
            n172 = call "Add State to Queue.vi"("State(s) In (\"\")"=w333) -> ("States Out"=w334:string)  [unwired: 14 in]
          }
          event "刷新按钮": Value Change {
            n173 = event-data() -> ()  [unwired: 1 in, 6 out]
            n174 = call "Add State to Queue.vi"("State(s) In (\"\")"=w340) -> ("States Out"=w339:string)  [unwired: 14 in]
            n175 = Two Button Dialog(message="请再次确实是否恢复出厂设置！" ("消息")) -> (T button?=w337:bool)  [unwired: 2 in]
            n176 = case shown="真" w337 {
              frame False {
              }
              frame True {
                w341 = u16 33 items=["Factory Reset"=33] ("数值")
                n177 = global read "多参数全局变量.vi" "MB session in"() -> (w342:refnum<class "MB_Master.lvclass">)
                n178 = call "0026H_浊度_命令寄存器写入.vi"("数值"=w341, "MB session in"=w342) -> ()  [unwired: 8 in, 2 out]
              }
            }
          }
          event "校准启动": Value Change {
            n179 = event-data() -> ()  [unwired: 1 in, 6 out]
            n180 = global read "多参数全局变量.vi" "校准运行状态"() -> (w344:T7)
            n181 = Bundle By Name(cluster=w344, "Turb"=TRUE) -> (w345:T7)
            n182 = global write "多参数全局变量.vi" "校准运行状态"(w345) -> ()
            n183 = call "Add State to Queue.vi"("State(s) In (\"\")"=w349, "State(s) At Back (\"\")"="init: all\nCal: Place standard solution\n Cal: Calibration process\nidle" ("State(s) In (\"\")")) -> ("States Out"=w348:string)  [unwired: 13 in]
          }
          event "校准停止": Value Change {
            n184 = event-data() -> ()  [unwired: 1 in, 6 out]
            n185 = call "Add State to Queue.vi"("State(s) In (\"\")"="init: all\nCal: Over\nidle" ("State(s) In (\"\")")) -> ("States Out"=w351:string)  [unwired: 14 in]
          }
        }
      }
    }
  }
  n186 = while {
    stop <- FALSE stop-if-true
    n187 = global read "多参数全局变量.vi" "权限"() -> (w356:enum16{"一级权限", "二级权限", "三级权限"})
    n188 = Wait (ms)(milliseconds to wait=u32 1000 ("等待时间（毫秒）")) -> ()  [unwired: 1 out]
    n189 = Not Equal?(x=w356, y=enum16{"一级权限", "二级权限", "三级权限"}."一级权限") -> (x != y?=w353:bool)
    n190 = property on="滤波设定" class="DigNum (严格)"("Visible"=w353) -> ()  [unwired: 2 in, 2 out]
    n191 = property on="偏移值补偿" class="DigNum (严格)"("Visible"=w353) -> ()  [unwired: 2 in, 2 out]
  }
